vi "Copy Library into Project.vi"(0 "Project":refnum<vi>, 5 "Library Path":path, 7 "Destination Folder":path, 9 "New TLB Name":string, 11 "error in":errorcluster) -> (15 "error out":errorcluster)   [LabVIEW 2014, in "TLB` Springboard.lvlib"]
uses:
  TLB` Springboard.lvlib
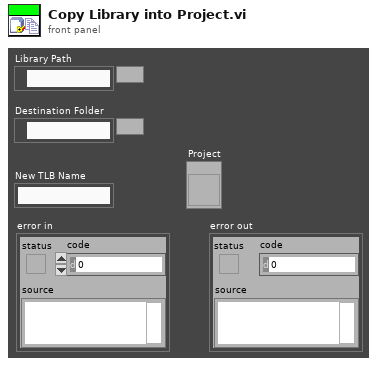
[diagram p1: front panel]
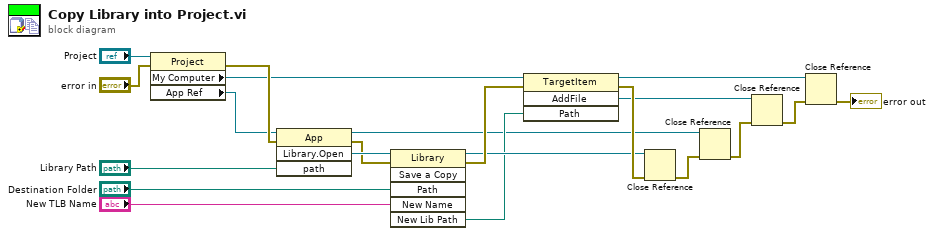
[diagram p0: block diagram]
diagram:
  n1 = property class="Project"(reference="Project", error in="error in") -> (error out=w21:errorcluster, "My Computer"=w6:refnum<vi>, "App Ref"=w18:refnum<vi>)  [unwired: 1 out]
  n2 = invoke class="App" method="Library.Open"(reference=w18, error in=w21, "path"="Library Path") -> (reference out=w3:refnum<vi>, error out=w4:errorcluster, "Open Library"=w9:refnum<vi>)  [unwired: 1 in, 1 out]
  n3 = invoke class="Library" method="Save a Copy"(reference=w9, error in=w4, "Path"="Destination Folder", "New Name"="New TLB Name") -> (reference out=w11:refnum<vi>, error out=w20:errorcluster, "New Lib Path"=w8:path)  [unwired: 2 in, 3 out]
  n4 = invoke class="TargetItem" method="AddFile"(reference=w6, error in=w20, "Path"=w8) -> (reference out=w12:refnum<vi>, error out=w16:errorcluster, "AddFile"=w13:refnum<vi>)  [unwired: 1 in, 1 out]
  n5 = Close Reference(reference=w11, error in (no error)=w16) -> (error out=w2:errorcluster)
  n6 = Close Reference(reference=w3, error in (no error)=w2) -> (error out=w1:errorcluster)
  n7 = Close Reference(reference=w13, error in (no error)=w1) -> (error out=w14:errorcluster)
  n8 = Close Reference(reference=w12, error in (no error)=w14) -> (error out=→"error out":errorcluster)
